vi "top_level_folder_location.vi"() -> (3 "Parent Folder":path)   [LabVIEW 2015]
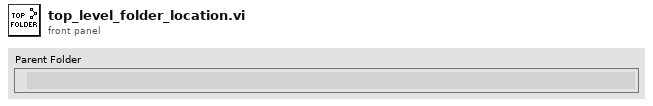
[diagram p1: front panel]
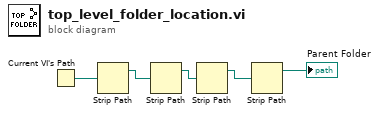
[diagram p0: block diagram]
diagram:
  n1 = Current VI's Path() -> (path=w5:path)
  n2 = Strip Path(path=w5) -> (stripped path=w4:path)  [unwired: 1 out]
  n3 = Strip Path(path=w4) -> (stripped path=w3:path)  [unwired: 1 out]
  n4 = Strip Path(path=w3) -> (stripped path=w2:path)  [unwired: 1 out]
  n5 = Strip Path(path=w2) -> (stripped path=→"Parent Folder":path)  [unwired: 1 out]
